vi "Get Engine Stream Filter IDs.vi"(7 "Ignore Error Arb ID?":bool=TRUE, 8 "error in (no error)":errorcluster, 11 "Refs":T1 {"Termination" items=["Off", "On"]}) -> (0 "error out":errorcluster, 2 "IDs":u32[](array[numeric]))   [LabVIEW 2019, in "CAN Streaming Support Engine.lvlib"]
uses:
  Diagnostics-Custom-Device/Source/SubModules/CAN-Streaming-Support/Addon/Addon Engine/CAN Streaming Support Engine.lvlib
  Types/Engine Stream API Refs.ctl
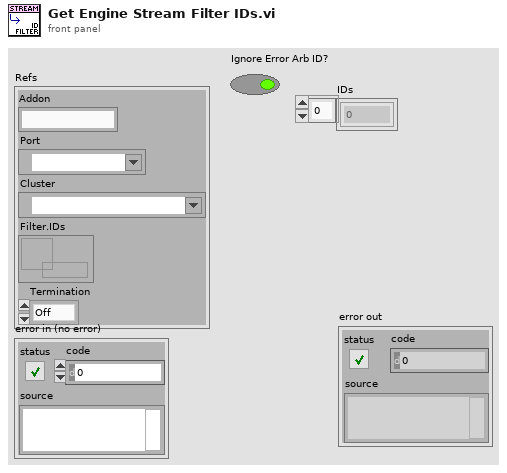
[diagram p1: front panel]
types:
  T1 = typedef "CAN Streaming Support Engine.lvlib/Engine Stream API Refs.ctl" = cluster{"Addon":string, "Port":refnum<k21>, "Cluster":refnum<k21>, "Filter.IDs":refnum<data-value>, "Termination":u32}
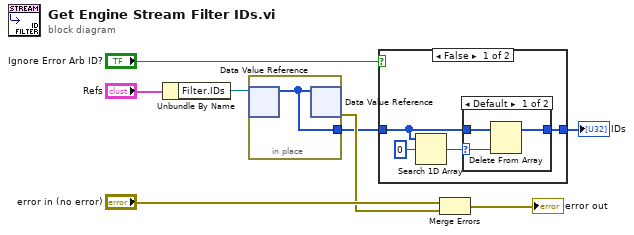
[diagram p0: block diagram]
diagram:
  n1 = Unbundle By Name("Refs") -> ("Filter.IDs"=w7:refnum<data-value>)
  n2 = in-place {
    in-place-border: [w9] -> w3
    n3 = in-place-dvr #1(w7) -> (w9:u32[])  [unwired: 1 out]
    n4 = in-place-dvr #1(w9) -> (w4:errorcluster)  [unwired: 1 out]
  }
  n5 = case shown="False" "Ignore Error Arb ID?" {
    tunnel: w3 -> [w11 w18]
    tunnel: [w10 w18] -> w2
    frame False {
      n6 = Search 1D Array(1D array=w11, element=u32 0) -> (index of element=w12:i32)  [unwired: 1 in]
      n7 = case shown="Default" w12 {
        selector: w12 -> [w14 _]
        tunnel: w11 -> [w16 w17]
        tunnel: [w15 w17] -> w10
        frame Default {
          n8 = Delete From Array(array=w16, index=w14) -> (array with subset deleted=w15:u32[])  [unwired: 1 in, 1 out]
        }
        frame -1 {
        }
      }
    }
    frame True {
    }
  }
  "IDs" <- w2
  n9 = Merge Errors("error in (no error)", w4) -> (→"error out":errorcluster)
